vi "gen MB frame -read device address.vi"() -> (3 "MB frame":string)   [LabVIEW 2016, in "MB _relays.lvlib"]
uses:
  MB _relays.lvlib
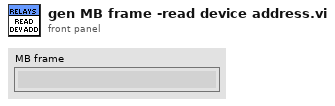
[diagram p1: front panel]
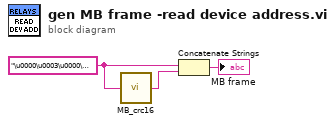
[diagram p0: block diagram]
diagram:
  w2 = "\u0000\u0003\u0000\u0000\u0000\u0001"
  n1 = call "MB_crc16.vi"("message"=w2) -> ("CRC16"=w3:string)  [unwired: 4 in]
  n2 = Concatenate Strings(w2, w3) -> (→"MB frame":string)
